vi "Filter Item.vi"(6 "Case Sensitive?":bool, 7 "Filter Type":T1, 8 "error in (no error)":errorcluster, 9 "Filter Value":string, 10 "Filter Column":T2, 11 "VI in":refnum<class "VI.lvclass">) -> (0 "error out":errorcluster, 2 "Include?":bool, 3 "VI out":refnum<class "VI.lvclass">)   [LabVIEW 2020, in "VI Properties Editor.lvlib" / "VI.lvclass"]
doc: "Checks whether <B>VI in</B> will be included in a filter defined by the other inputs."
uses:
  VI.lvclass
  C:/Users/acasalen/Documents/LabVIEW Data/Projects/VI-Properties-Editor/source/Classes/Item/Item.lvclass
  CTLs/Filter Column.ctl
  CTLs/Filter Type.ctl
  Control/Control.lvclass
  VI Properties Editor.lvlib
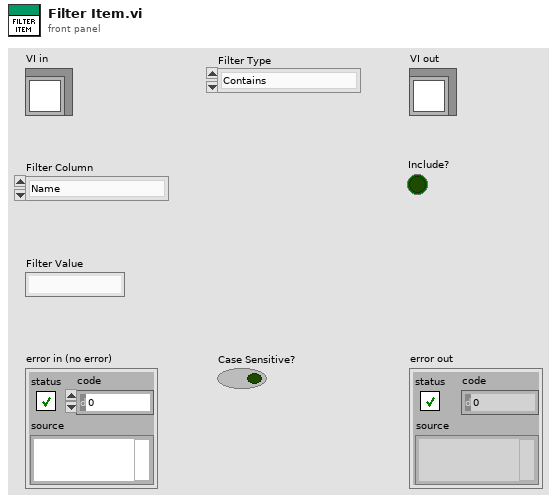
[diagram p1: front panel]
types:
  T1 = typedef "VI Properties Editor.lvlib/Filter Type.ctl" = enum16{"Contains", "Equals", "Starts with", "Ends with", "Is empty", "Does not contain", "Does not equal", "Is not empty"}
  T2 = typedef "VI Properties Editor.lvlib/Filter Column.ctl" = enum16{"Name", "Path", "Type", "Window Title", "Description", "Help Path", "Help Tag", "Custom Title?", "Reentrancy", "Inlined?", "Help URL", "Help Type", "Allow Debugging?", "Auto Error Handling?", "Run When Opened?", "Suspend When Called?", "Priority", "Preferred Exec Sytem", "Control Label", "Control Caption", "Control Description", "Control Tip Strip"}
  T3 = enum32{"invalid VI type", "Standard VI", "Control VI", "Global VI", "Polymorphic VI", "Configuration VI", "SubSystem", "Facade VI", "Method VI", "Statechart Diagram VI"}
  T4 = enum16{"Share clones between instances", "Preallocate clone for each instance"}
  T5 = enum32{"invalid priority", "background priority", "normal priority", "above normal priority", "high priority", "time critical priority", "subroutine"}
  T6 = enum32{"invalid execution system", "user interface", "standard", "instrument i/o", "data acquisition", "other 1", "other 2", "same as caller"}
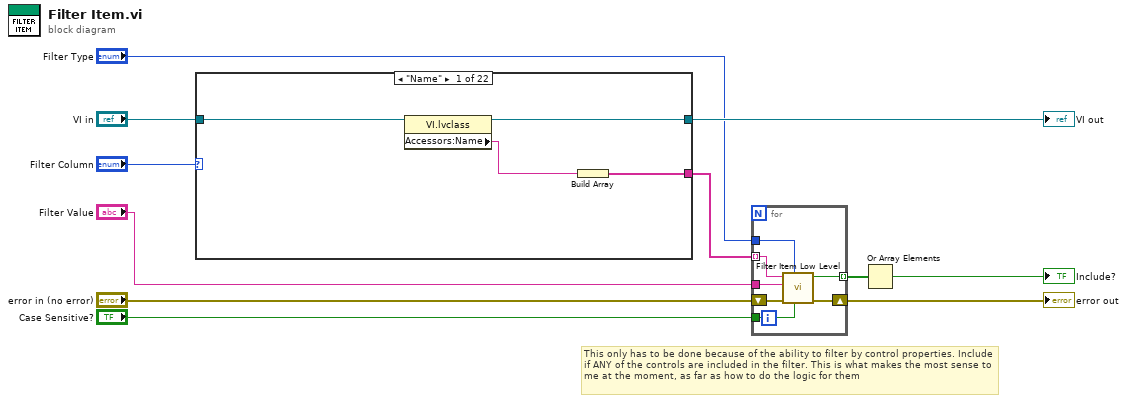
[diagram p0: block diagram]
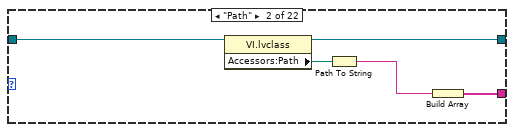
[diagram p2: hidden frame]
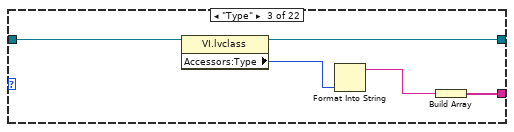
[diagram p3: hidden frame]
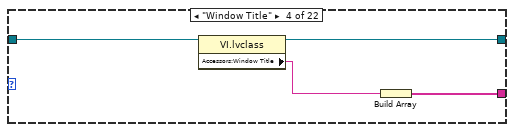
[diagram p4: hidden frame]
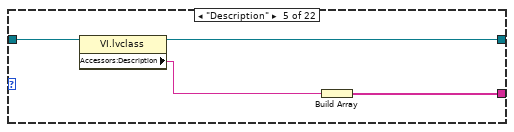
[diagram p5: hidden frame]
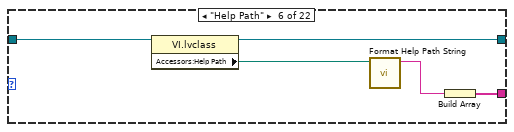
[diagram p6: hidden frame]
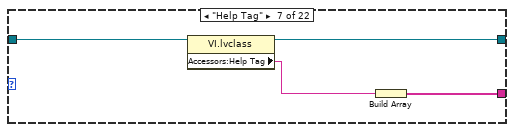
[diagram p7: hidden frame]
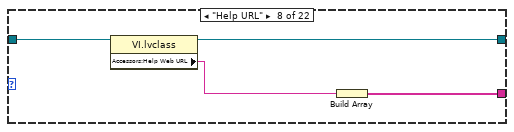
[diagram p8: hidden frame]
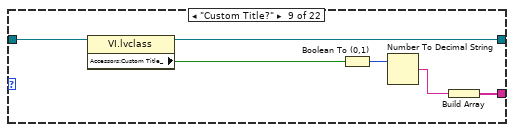
[diagram p9: hidden frame]
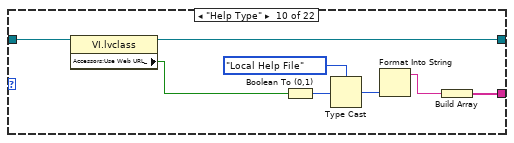
[diagram p10: hidden frame]
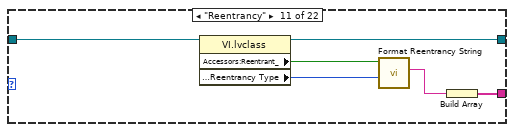
[diagram p11: hidden frame]
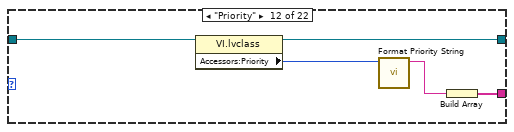
[diagram p12: hidden frame]
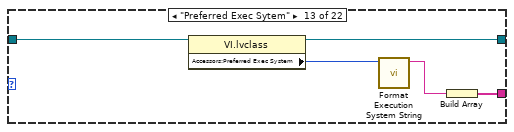
[diagram p13: hidden frame]
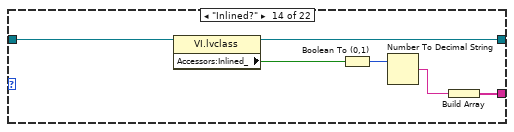
[diagram p14: hidden frame]
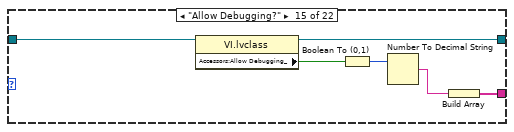
[diagram p15: hidden frame]
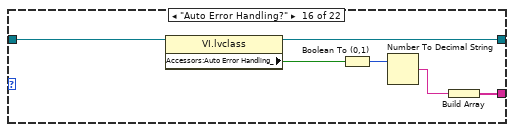
[diagram p16: hidden frame]
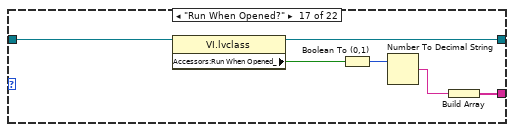
[diagram p17: hidden frame]
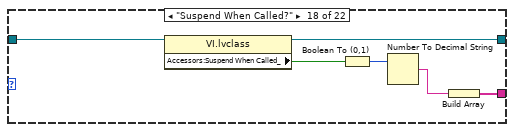
[diagram p18: hidden frame]
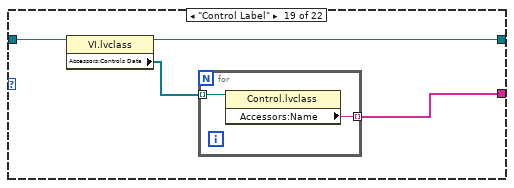
[diagram p19: hidden frame]
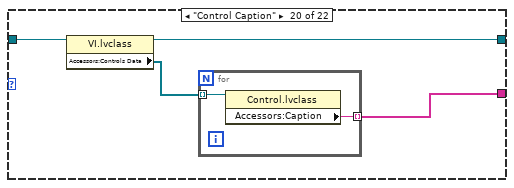
[diagram p20: hidden frame]
diagram:
  # "This only has to be done because of the ability to filter by control properties. Include if ANY of the controls are included in the filter. This is what makes the most sense to me at the moment, as far as how to do the logic for them"
  n1 = case shown="\"Name\"" "Filter Column" {
    tunnel: [w12 w16 w21 w26 w30 w34 w39 w43 w47 w53 w61 w67 w72 w77 w83 w89 w95 w101 w107 w113 w119 w125] -> w6
    tunnel: "VI in" -> [w15 w19 w24 w29 w33 w37 w42 w46 w50 w57 w65 w70 w75 w80 w86 w92 w98 w104 w110 w116 w122 w128]
    tunnel: [w14 w18 w23 w28 w32 w35 w41 w45 w49 w55 w62 w69 w74 w79 w85 w90 w96 w103 w109 w115 w121 w127] -> w10
    frame "Name" {
      n2 = property class="VI.lvclass"(reference=w15) -> (reference out=w14:refnum<class "VI.lvclass">, "Accessors:Name"=w13:string)  [unwired: 1 in, 1 out]
      n3 = Build Array(w13) -> (w12:string[])
    }
    frame "Path" {
      n4 = property class="VI.lvclass"(reference=w19) -> (reference out=w18:refnum<class "VI.lvclass">, "Accessors:Path"=w17:path)  [unwired: 1 in, 1 out]
      n5 = Path To String(path=w17) -> (string=w20:string)
      n6 = Build Array(w20) -> (w16:string[])
    }
    frame "Type" {
      n7 = property class="VI.lvclass"(reference=w24) -> (reference out=w23:refnum<class "VI.lvclass">, "Accessors:Type"=w22:T3)  [unwired: 1 in, 1 out]
      n8 = Format Into String(w22) -> (resulting string=w25:string)  [unwired: 3 in, 1 out]
      n9 = Build Array(w25) -> (w21:string[])
    }
    frame "Window Title" {
      n10 = property class="VI.lvclass"(reference=w29) -> (reference out=w28:refnum<class "VI.lvclass">, "Accessors:Window Title"=w27:string)  [unwired: 1 in, 1 out]
      n11 = Build Array(w27) -> (w26:string[])
    }
    frame "Description" {
      n12 = property class="VI.lvclass"(reference=w33) -> (reference out=w32:refnum<class "VI.lvclass">, "Accessors:Description"=w31:string)  [unwired: 1 in, 1 out]
      n13 = Build Array(w31) -> (w30:string[])
    }
    frame "Help Path" {
      n14 = property class="VI.lvclass"(reference=w37) -> (reference out=w35:refnum<class "VI.lvclass">, "Accessors:Help Path"=w36:path)  [unwired: 1 in, 1 out]
      n15 = call "Format Help Path String.vi"("Help Path"=w36) -> ("Help Path String"=w38:string)  [unwired: 10 in]
      n16 = Build Array(w38) -> (w34:string[])
    }
    frame "Help Tag" {
      n17 = property class="VI.lvclass"(reference=w42) -> (reference out=w41:refnum<class "VI.lvclass">, "Accessors:Help Tag"=w40:string)  [unwired: 1 in, 1 out]
      n18 = Build Array(w40) -> (w39:string[])
    }
    frame "Help URL" {
      n19 = property class="VI.lvclass"(reference=w46) -> (reference out=w45:refnum<class "VI.lvclass">, "Accessors:Help Web URL"=w44:string)  [unwired: 1 in, 1 out]
      n20 = Build Array(w44) -> (w43:string[])
    }
    frame "Custom Title?" {
      n21 = property class="VI.lvclass"(reference=w50) -> (reference out=w49:refnum<class "VI.lvclass">, "Accessors:Custom Title_"=w48:bool)  [unwired: 1 in, 1 out]
      n22 = Boolean To (0,1)(Boolean=w48) -> (0, 1=w52:i16)
      n23 = Number To Decimal String(number=w52) -> (decimal integer string=w51:string)  [unwired: 1 in]
      n24 = Build Array(w51) -> (w47:string[])
    }
    frame "Help Type" {
      n25 = property class="VI.lvclass"(reference=w57) -> (reference out=w55:refnum<class "VI.lvclass">, "Accessors:Use Web URL_"=w56:bool)  [unwired: 1 in, 1 out]
      n26 = Boolean To (0,1)(Boolean=w56) -> (0, 1=w60:i16)
      n27 = Type Cast(type=enum16{"Local Help File", "Web-based Help"}."Local Help File" ("FP.Help Type"), x=w60) -> (*(type *) &x=w58:enum16{"Local Help File", "Web-based Help"})
      n28 = Format Into String(w58) -> (resulting string=w54:string)  [unwired: 3 in, 1 out]
      n29 = Build Array(w54) -> (w53:string[])
    }
    frame "Reentrancy" {
      n30 = property class="VI.lvclass"(reference=w65) -> (reference out=w62:refnum<class "VI.lvclass">, "Accessors:Reentrant_"=w64:bool, "Accessors:Reentrancy Type"=w63:T4)  [unwired: 1 in, 1 out]
      n31 = call "Format Reentrancy String.vi"("Reentrancy Type"=w63, "Reentrant?"=w64) -> ("Reentrancy String"=w66:string)  [unwired: 9 in]
      n32 = Build Array(w66) -> (w61:string[])
    }
    frame "Priority" {
      n33 = property class="VI.lvclass"(reference=w70) -> (reference out=w69:refnum<class "VI.lvclass">, "Accessors:Priority"=w68:T5)  [unwired: 1 in, 1 out]
      n34 = call "Format Priority String.vi"("Priority"=w68) -> ("Priority String"=w71:string)  [unwired: 10 in]
      n35 = Build Array(w71) -> (w67:string[])
    }
    frame "Preferred Exec Sytem" {
      n36 = property class="VI.lvclass"(reference=w75) -> (reference out=w74:refnum<class "VI.lvclass">, "Accessors:Preferred Exec System"=w73:T6)  [unwired: 1 in, 1 out]
      n37 = call "Format Execution System String.vi"("Preferred Exec System"=w73) -> ("Preferred Exec System String"=w76:string)  [unwired: 10 in]
      n38 = Build Array(w76) -> (w72:string[])
    }
    frame "Inlined?" {
      n39 = property class="VI.lvclass"(reference=w80) -> (reference out=w79:refnum<class "VI.lvclass">, "Accessors:Inlined_"=w78:bool)  [unwired: 1 in, 1 out]
      n40 = Boolean To (0,1)(Boolean=w78) -> (0, 1=w82:i16)
      n41 = Number To Decimal String(number=w82) -> (decimal integer string=w81:string)  [unwired: 1 in]
      n42 = Build Array(w81) -> (w77:string[])
    }
    frame "Allow Debugging?" {
      n43 = property class="VI.lvclass"(reference=w86) -> (reference out=w85:refnum<class "VI.lvclass">, "Accessors:Allow Debugging_"=w84:bool)  [unwired: 1 in, 1 out]
      n44 = Boolean To (0,1)(Boolean=w84) -> (0, 1=w88:i16)
      n45 = Number To Decimal String(number=w88) -> (decimal integer string=w87:string)  [unwired: 1 in]
      n46 = Build Array(w87) -> (w83:string[])
    }
    frame "Auto Error Handling?" {
      n47 = property class="VI.lvclass"(reference=w92) -> (reference out=w90:refnum<class "VI.lvclass">, "Accessors:Auto Error Handling_"=w91:bool)  [unwired: 1 in, 1 out]
      n48 = Boolean To (0,1)(Boolean=w91) -> (0, 1=w94:i16)
      n49 = Number To Decimal String(number=w94) -> (decimal integer string=w93:string)  [unwired: 1 in]
      n50 = Build Array(w93) -> (w89:string[])
    }
    frame "Run When Opened?" {
      n51 = property class="VI.lvclass"(reference=w98) -> (reference out=w96:refnum<class "VI.lvclass">, "Accessors:Run When Opened_"=w97:bool)  [unwired: 1 in, 1 out]
      n52 = Boolean To (0,1)(Boolean=w97) -> (0, 1=w100:i16)
      n53 = Number To Decimal String(number=w100) -> (decimal integer string=w99:string)  [unwired: 1 in]
      n54 = Build Array(w99) -> (w95:string[])
    }
    frame "Suspend When Called?" {
      n55 = property class="VI.lvclass"(reference=w104) -> (reference out=w103:refnum<class "VI.lvclass">, "Accessors:Suspend When Called_"=w102:bool)  [unwired: 1 in, 1 out]
      n56 = Boolean To (0,1)(Boolean=w102) -> (0, 1=w106:i16)
      n57 = Number To Decimal String(number=w106) -> (decimal integer string=w105:string)  [unwired: 1 in]
      n58 = Build Array(w105) -> (w101:string[])
    }
    frame "Control Label" {
      n59 = property class="VI.lvclass"(reference=w110) -> (reference out=w109:refnum<class "VI.lvclass">, "Accessors:Controls Data"=w108:refnum<class "Control.lvclass">[])  [unwired: 1 in, 1 out]
      n60 = for {
        tunnel: w108 -> [w112] mode=indexing
        tunnel: [w111] -> w107 mode=indexing
        n61 = property class="Control.lvclass"(reference=w112) -> ("Accessors:Name"=w111:string)  [unwired: 1 in, 2 out]
      }
    }
    frame "Control Caption" {
      n62 = property class="VI.lvclass"(reference=w116) -> (reference out=w115:refnum<class "VI.lvclass">, "Accessors:Controls Data"=w114:refnum<class "Control.lvclass">[])  [unwired: 1 in, 1 out]
      n63 = for {
        tunnel: w114 -> [w118] mode=indexing
        tunnel: [w117] -> w113 mode=indexing
        n64 = property class="Control.lvclass"(reference=w118) -> ("Accessors:Caption"=w117:string)  [unwired: 1 in, 2 out]
      }
    }
    frame "Control Description" {
      n65 = property class="VI.lvclass"(reference=w122) -> (reference out=w121:refnum<class "VI.lvclass">, "Accessors:Controls Data"=w120:refnum<class "Control.lvclass">[])  [unwired: 1 in, 1 out]
      n66 = for {
        tunnel: w120 -> [w124] mode=indexing
        tunnel: [w123] -> w119 mode=indexing
        n67 = property class="Control.lvclass"(reference=w124) -> ("Accessors:Description"=w123:string)  [unwired: 1 in, 2 out]
      }
    }
    frame "Control Tip Strip" {
      n68 = property class="VI.lvclass"(reference=w128) -> (reference out=w127:refnum<class "VI.lvclass">, "Accessors:Controls Data"=w126:refnum<class "Control.lvclass">[])  [unwired: 1 in, 1 out]
      n69 = for {
        tunnel: w126 -> [w130] mode=indexing
        tunnel: [w129] -> w125 mode=indexing
        n70 = property class="Control.lvclass"(reference=w130) -> ("Accessors:Tip Strip"=w129:string)  [unwired: 1 in, 2 out]
      }
    }
  }
  "VI out" <- w10
  n71 = for {
    shift-right: [w136] -> w8
    shift-left: "error in (no error)" -> [w137]
    tunnel: w6 -> [w134] mode=indexing
    tunnel: "Filter Value" -> [w135]
    tunnel: "Filter Type" -> [w133]
    tunnel: [w132] -> w1 mode=indexing
    tunnel: "Case Sensitive?" -> [w131]
    n72 = call "Filter Item Low Level.vi"("Case Sensitive?"=w131, "Filter Type"=w133, "error in (no error)"=w137, "Filter Value"=w135, "Item Value"=w134) -> ("error out"=w136:errorcluster, "Include?"=w132:bool)  [unwired: 5 in]
  }
  "error out" <- w8
  n73 = Or Array Elements(Boolean array=w1) -> (logical OR=→"Include?":bool)
